vi "teste.vi"() -> ()   [LabVIEW 2014]
panel:
  out "x+y":dbl
  in  "y":dbl
  in  "Numeric Control":dbl
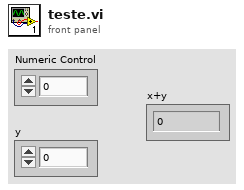
[diagram p1: front panel]
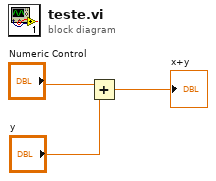
[diagram p0: block diagram]
diagram:
  n1 = Add(x="Numeric Control", y="y") -> (x+y=→"x+y":dbl)
